vi "Expt-7_Array-operations.vi"() -> ()   [LabVIEW 2020]
panel:
  out "Array while":dbl[](array[numeric])
  out "Array 2":dbl[][](array[numeric])
  out "Array output":dbl[][](array[numeric])
  in  "Columns":i32
  in  "Rows":i32
  out "current time":timestamp
  out "min value":dbl
  out "max value":dbl
  in  "Input array":dbl[](array[numeric])
  in  "stop":bool
  out "Array for":dbl[](array[numeric])
  out "Even numbers":i32[](array[numeric])
  in  "Number of even numbers":i32
  in  "Number of random numbers":i32
  # "1)(a)"
  # "1)(b)"
  # "2)(a)"
  # "2)(b)"
  # "3)"
  # "4)"
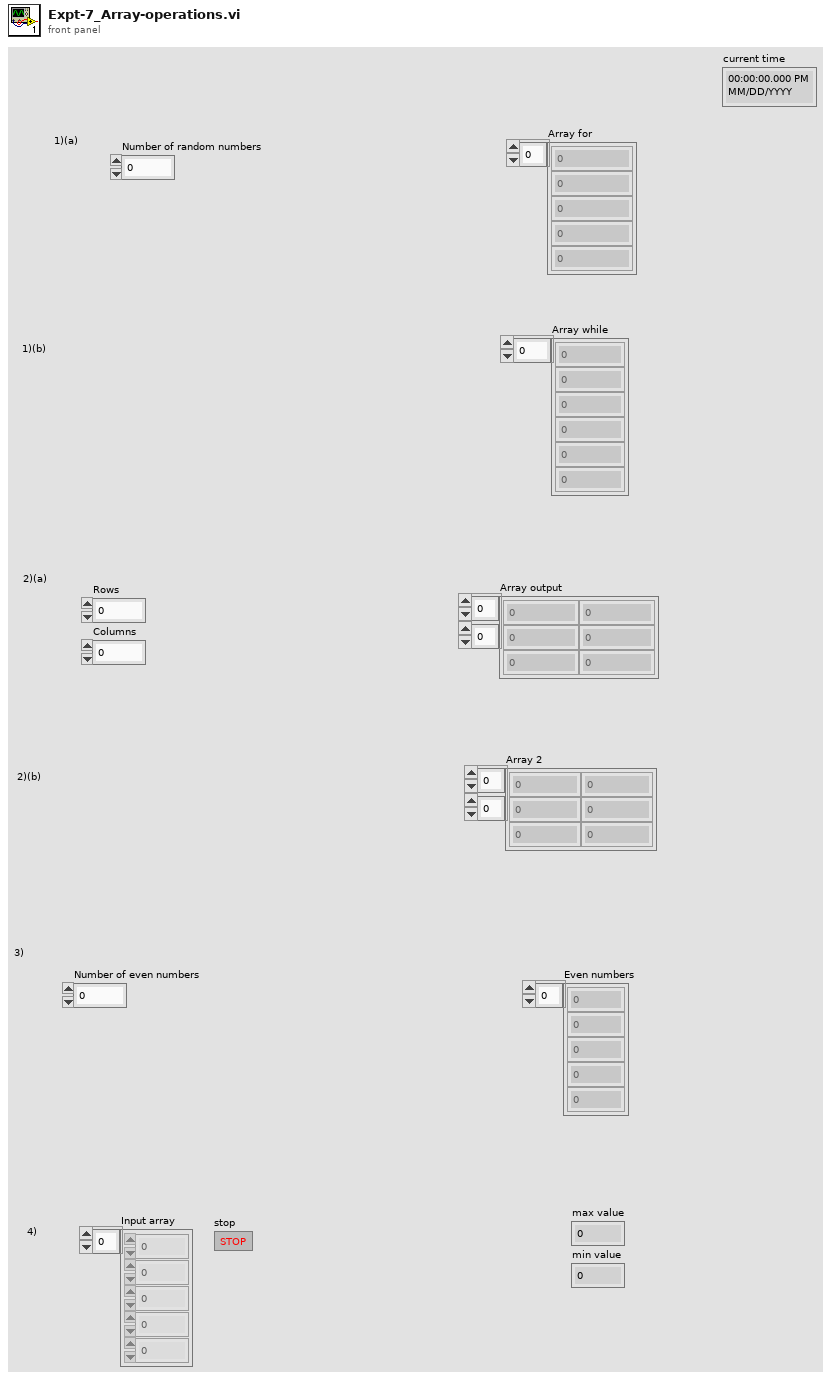
[diagram p1: front panel]
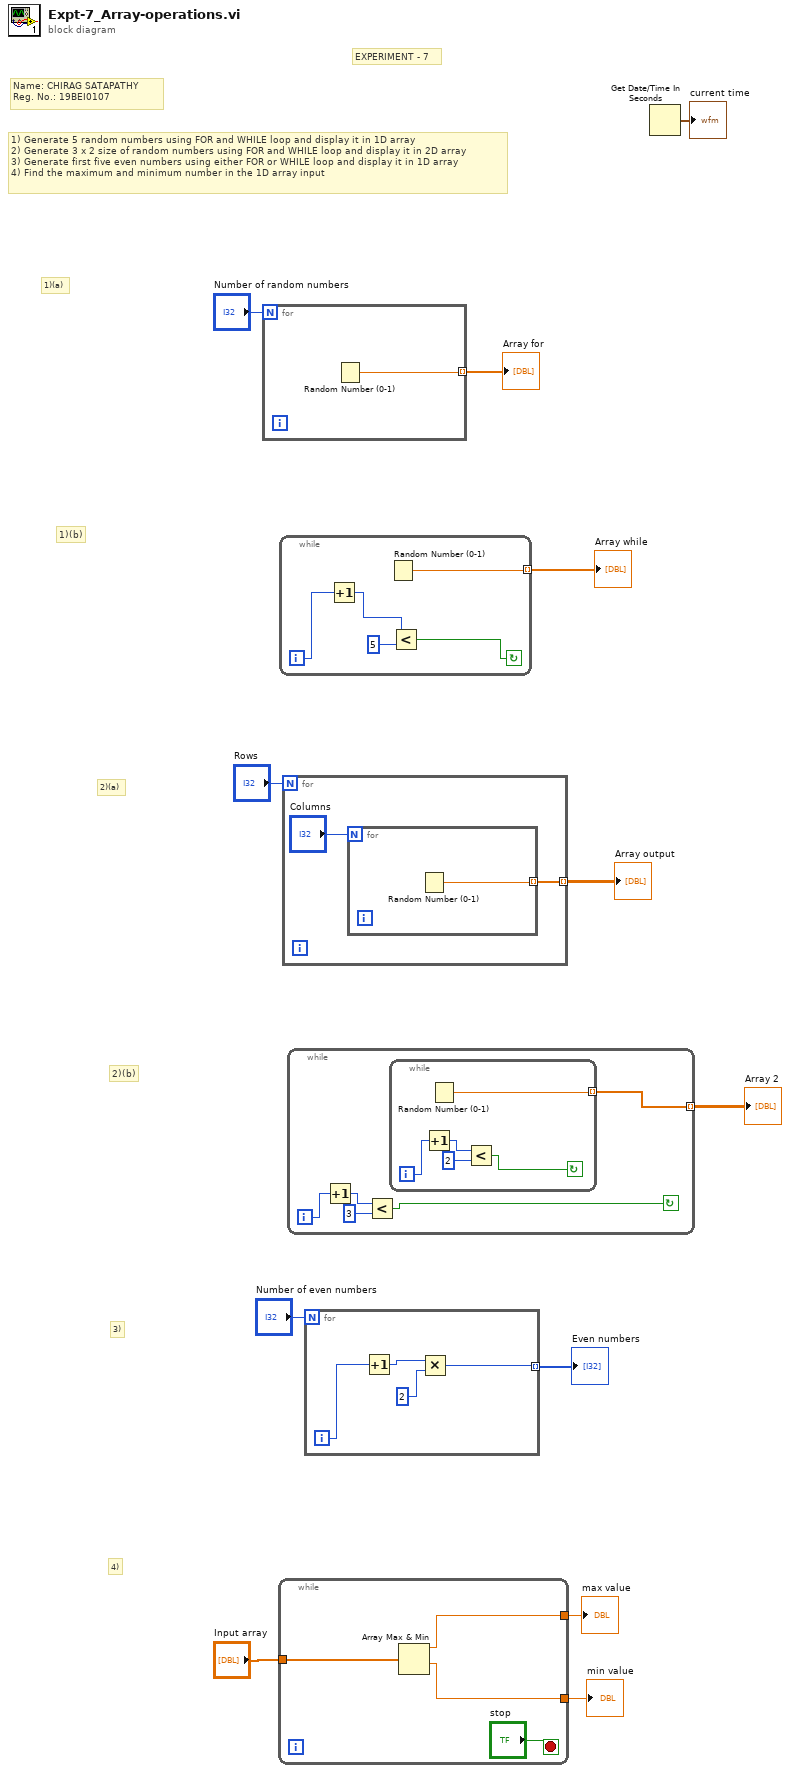
[diagram p0: block diagram]
diagram:
  # "2)(b)"
  # "1)(b)"
  # "2)(a)"
  # "4)"
  # "3)"
  # "1)(a)"
  # "Name: CHIRAG SATAPATHY\nReg. No.: 19BEI0107"
  # "EXPERIMENT - 7"
  # "1) Generate 5 random numbers using FOR and WHILE loop and display it in 1D array\n2) Generate 3 x 2 size of random numbers using FOR and WHILE loop and display it in 2D array\n3) Generate first five even numbers using either FOR or WHILE loop and display it in 1D array\n4) Find the maximum and minimum number in the 1D array input"
  n1 = for {
    N: "Number of random numbers" -> [_]
    tunnel: [w13] -> w9 mode=indexing
    n2 = Random Number (0-1)() -> (number: 0 to 1=w13:dbl)
  }
  "Array for" <- w9
  n3 = while {
    tunnel: "Input array" -> [w16]
    tunnel: [w15] -> w7
    tunnel: [w14] -> w6
    stop <- "stop" stop-if-true
    n4 = Array Max & Min(array=w16) -> (max value=w15:dbl, min value=w14:dbl)  [unwired: 2 out]
  }
  "max value" <- w7
  "min value" <- w6
  n5 = while {
    tunnel: [w19] -> w1 mode=indexing
    i -> [w22]
    stop <- w20 continue-if-true
    n6 = Increment(x=w22) -> (x+1=w21:i32)
    n7 = Random Number (0-1)() -> (number: 0 to 1=w19:dbl)
    n8 = Less?(x=w21, y=5) -> (x < y?=w20:bool)
  }
  "Array while" <- w1
  n9 = for {
    N: "Rows" -> [_]
    tunnel: [w23] -> w3 mode=indexing
    n10 = for {
      N: "Columns" -> [_]
      tunnel: [w25] -> w23 mode=indexing
      n11 = Random Number (0-1)() -> (number: 0 to 1=w25:dbl)
    }
  }
  "Array output" <- w3
  n12 = while {
    tunnel: [w30] -> w2 mode=indexing
    i -> [w29]
    stop <- w26 continue-if-true
    n13 = Increment(x=w29) -> (x+1=w28:i32)
    n14 = Less?(x=w28, y=3) -> (x < y?=w26:bool)
    n15 = while {
      tunnel: [w35] -> w30 mode=indexing
      i -> [w32]
      stop <- w31 continue-if-true
      n16 = Increment(x=w32) -> (x+1=w34:i32)
      n17 = Random Number (0-1)() -> (number: 0 to 1=w35:dbl)
      n18 = Less?(x=w34, y=2) -> (x < y?=w31:bool)
    }
  }
  "Array 2" <- w2
  n19 = for {
    N: "Number of even numbers" -> [_]
    tunnel: [w36] -> w10 mode=indexing
    i -> [w39]
    n20 = Increment(x=w39) -> (x+1=w38:i32)
    n21 = Multiply(x=w38, y=2) -> (x*y=w36:i32)
  }
  "Even numbers" <- w10
  n22 = Get Date/Time In Seconds() -> (seconds since 1Jan1904=→"current time":timestamp)
